vi "Replace Wheels in Steering Frame.vi"   [LabVIEW 2017, in "NI_Robotics_Steering Frame.lvclass"]
doc: "Replaces wheels in <B>steering frame in</B> with the wheels you specify. You must manually select the polymorphic instance to use."
uses:
  <vilib>/robotics/Steering/Steering Frame/NI_Robotics_Steering Frame.lvclass
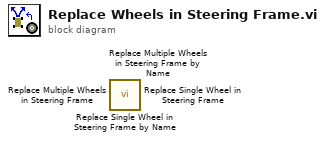
[diagram p0: block diagram]
diagram:
  n1 = call <vilib>:"Replace Single Wheel in Steering Frame by Name.vi"() -> ()  [unwired: 9 in, 3 out]
  n2 = call <vilib>:"Replace Multiple Wheels in Steering Frame by Name.vi"() -> ()  [unwired: 9 in, 3 out]
  n3 = call <vilib>:"Replace Multiple Wheels in Steering Frame.vi"() -> ()  [unwired: 9 in, 3 out]
  n4 = call <vilib>:"Replace Single Wheel in Steering Frame.vi"() -> ()  [unwired: 9 in, 3 out]
